vi "FW_search_results_array.vi"(11 "frames_Result":T1[](array[typedef])) -> (3 "Waveform Graph":sgl[][](graph))   [LabVIEW 2021, in "Framework_lib.lvlib"]
uses:
  QMH/Framework_lib.lvlib
  FW_Frames_Data.ctl
  QMH/QMH_Producer_type.ctl
  FW_Image_resultant_data.ctl
  <vilib>/vision/Image Controls.llb/IMAQ Image.ctl
  QMH/QMH_references_enum.ctl
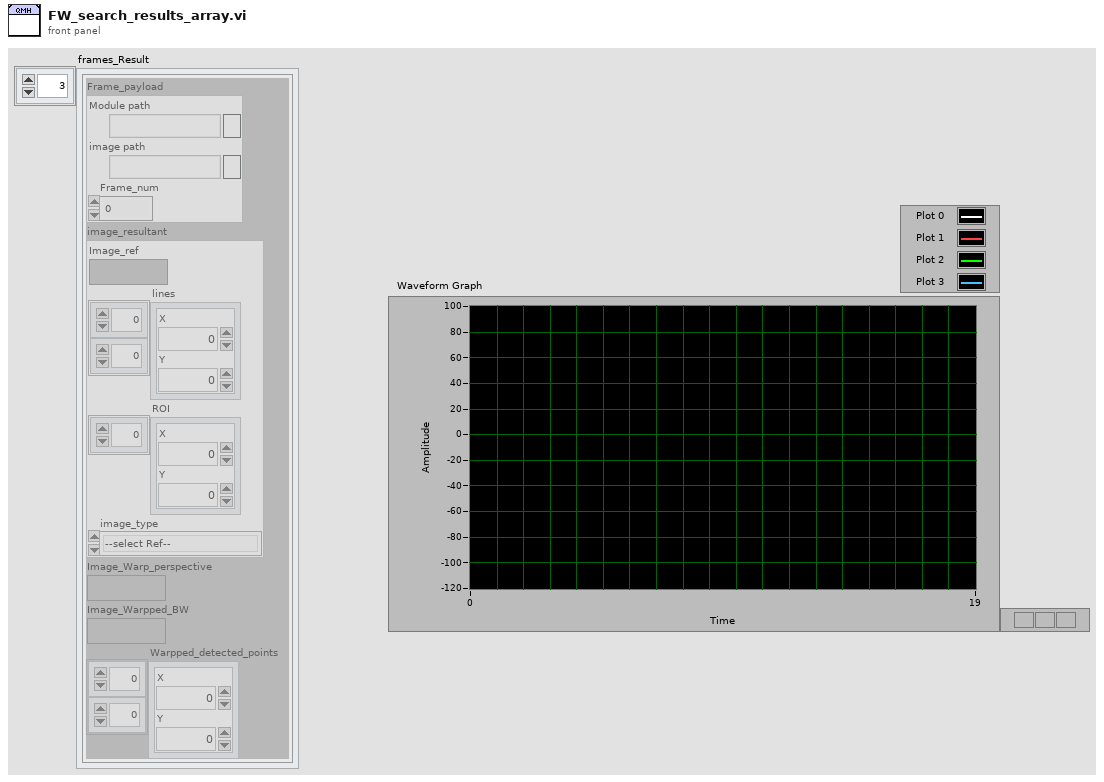
[diagram p1: front panel]
types:
  T1 = typedef "Framework_lib.lvlib/FW_Frames_Data.ctl" = cluster{"Frame_payload":T2, "image_resultant":T3, "Image_Warp_perspective":T4, "Image_Warpped_BW":T4, "Warpped_detected_points":cluster{"X":sgl, "Y":sgl}[][]}
  T2 = typedef "Framework_lib.lvlib/QMH_Producer_type.ctl" = cluster{"Module path":path, "image path":path, "Frame_num":u16}
  T3 = typedef "Framework_lib.lvlib/FW_Image_resultant_data.ctl" = cluster{"Image_ref":T4, "lines":cluster{"X":dbl, "Y":dbl}[][], "ROI":cluster{"X":dbl, "Y":dbl}[], "image_type":T5}
  T4 = typedef "IMAQ Image.ctl" = refnum<image>
  T5 = typedef "Framework_lib.lvlib/QMH_references_enum.ctl" = enum16{"--select Ref--", "Consumer_SUT", "Consumer_Annot", "Compute_Results"}
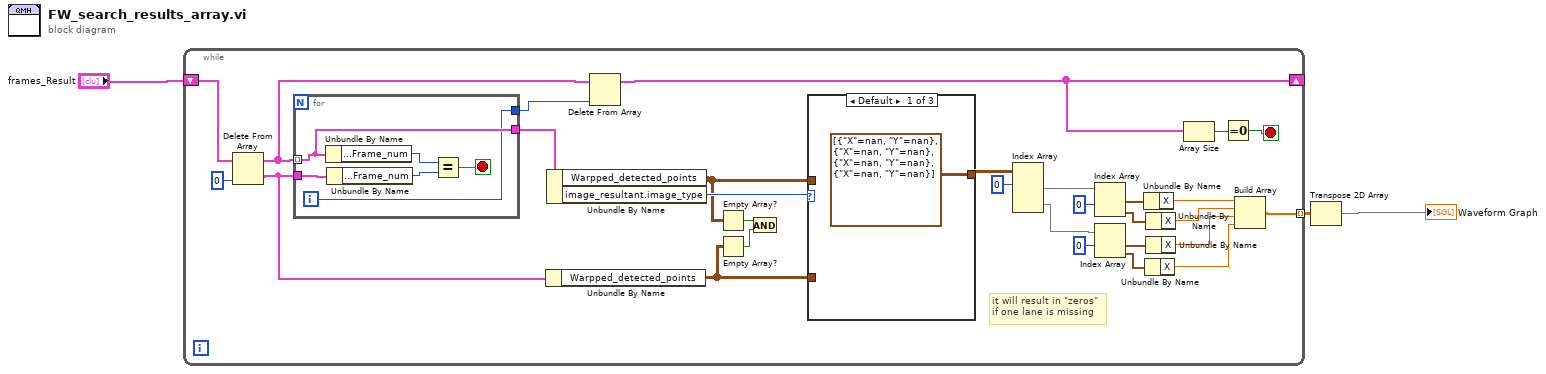
[diagram p0: block diagram]
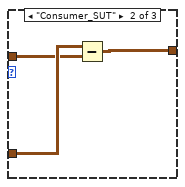
[diagram p2: hidden frame]
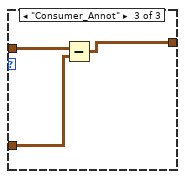
[diagram p3: hidden frame]
diagram:
  n1 = while {
    shift-right: [w25] -> _
    shift-left: "frames_Result" -> [w31]
    tunnel: [w8] -> w2 mode=indexing
    stop <- w23 stop-if-true
    # "it will result in \"zeros\"\nif one lane is missing"
    n2 = Delete From Array(array=w31, index=0) -> (deleted portion=w28:T1, array with subset deleted=w26:T1[])  [unwired: 1 in]
    n3 = for {
      tunnel: w28 -> [w45]
      tunnel: w26 -> [w41] mode=indexing
      tunnel: [w41] -> w30
      tunnel: [w40] -> w27
      i -> [w40]
      stop <- w42 stop-if-true
      n4 = Unbundle By Name(w41) -> ("Frame_payload.Frame_num"=w43:u16)
      n5 = Unbundle By Name(w45) -> ("Frame_payload.Frame_num"=w44:u16)
      n6 = Equal?(x=w43, y=w44) -> (x = y?=w42:bool)
    }
    n7 = Unbundle By Name(w28) -> ("Warpped_detected_points"=w7:cluster{"X":sgl, "Y":sgl}[][])
    n8 = Unbundle By Name(w30) -> ("Warpped_detected_points"=w6:cluster{"X":sgl, "Y":sgl}[][], "image_resultant.image_type"=w29:T5)
    n9 = Delete From Array(array=w26, index=w27) -> (array with subset deleted=w25:T1[])  [unwired: 1 in, 1 out]
    n10 = Empty Array?(array=w6) -> (empty?=w5:bool)
    n11 = Empty Array?(array=w7) -> (empty?=w4:bool)
    n12 = And(x=w5, y=w4) -> ()  [unwired: 1 out]
    n13 = case shown="Default" w29 {
      tunnel: w7 -> [_ w36 w38]
      tunnel: w6 -> [_ w35 w39]
      tunnel: [cluster{"X":sgl, "Y":dbl}[][] [[{"X"=nan, "Y"=nan}, {"X"=nan, "Y"=nan}], [{"X"=nan, "Y"=nan}, {"X"=nan, "Y"=nan}]] w34 w37] -> w22
      frame Default {
      }
      frame "Consumer_SUT" {
        n14 = Subtract(x=w36, y=w35) -> (x-y=w34:cluster{"X":sgl, "Y":sgl}[][])
      }
      frame "Consumer_Annot" {
        n15 = Subtract(x=w39, y=w38) -> (x-y=w37:cluster{"X":sgl, "Y":sgl}[][])
      }
    }
    n16 = Index Array(array=w22, index (row) #1=0 ("index (row)")) -> (element #1=w20:cluster{"X":sgl, "Y":dbl}[], element #2=w17:cluster{"X":sgl, "Y":dbl}[])  [unwired: 3 in]
    n17 = Index Array(array=w20, index #1=0 ("index")) -> (element #1=w16:cluster{"X":sgl, "Y":dbl}, element #2=w15:cluster{"X":sgl, "Y":dbl})  [unwired: 1 in]
    n18 = Index Array(array=w17, index #1=0 ("index")) -> (element #1=w13:cluster{"X":sgl, "Y":dbl}, element #2=w14:cluster{"X":sgl, "Y":dbl})  [unwired: 1 in]
    n19 = Unbundle By Name(w16) -> ("X"=w12:sgl)
    n20 = Unbundle By Name(w14) -> ("X"=w9:sgl)
    n21 = Unbundle By Name(w15) -> ("X"=w11:sgl)
    n22 = Unbundle By Name(w13) -> ("X"=w10:sgl)
    n23 = Array Size(array=w25) -> (size(s)=w24:i32)
    n24 = Equal To 0?(x=w24) -> (x = 0?=w23:bool)
    n25 = Build Array(w12, w11, w10, w9) -> (w8:sgl[])
  }
  n26 = Transpose 2D Array(2D array=w2) -> (transposed array=→"Waveform Graph":sgl[][])
